vi "Periodic Tasks.vi"(8 "error in":errorcluster) -> ()   [LabVIEW 2018]
doc: "This VI runs in parallel to other robot code. It can contain as many user-defined periodic loops as you need. These can carry out PID or other sorts of timed response."
uses:
  <vilib>/Rock Robotics/Network Tables/NT Write Boolean.vi
  <vilib>/Rock Robotics/Network Tables/NT Write Number.vi
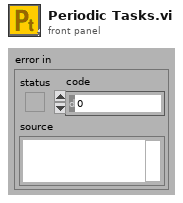
[diagram p1: front panel]
types:
  T1 = typedef "WPI_AnalogChannelDevRef.ctl" = cluster{"DevStatus":errorcluster, "Analog Channel":T2}
  T2 = typedef "FPGA_AIChannel.ctl" = enum8{"AI 0", "AI 1", "AI 2", "AI 3", "AI MXP 0", "AI MXP 1", "AI MXP 2", "AI MXP 3", "Invalid"}
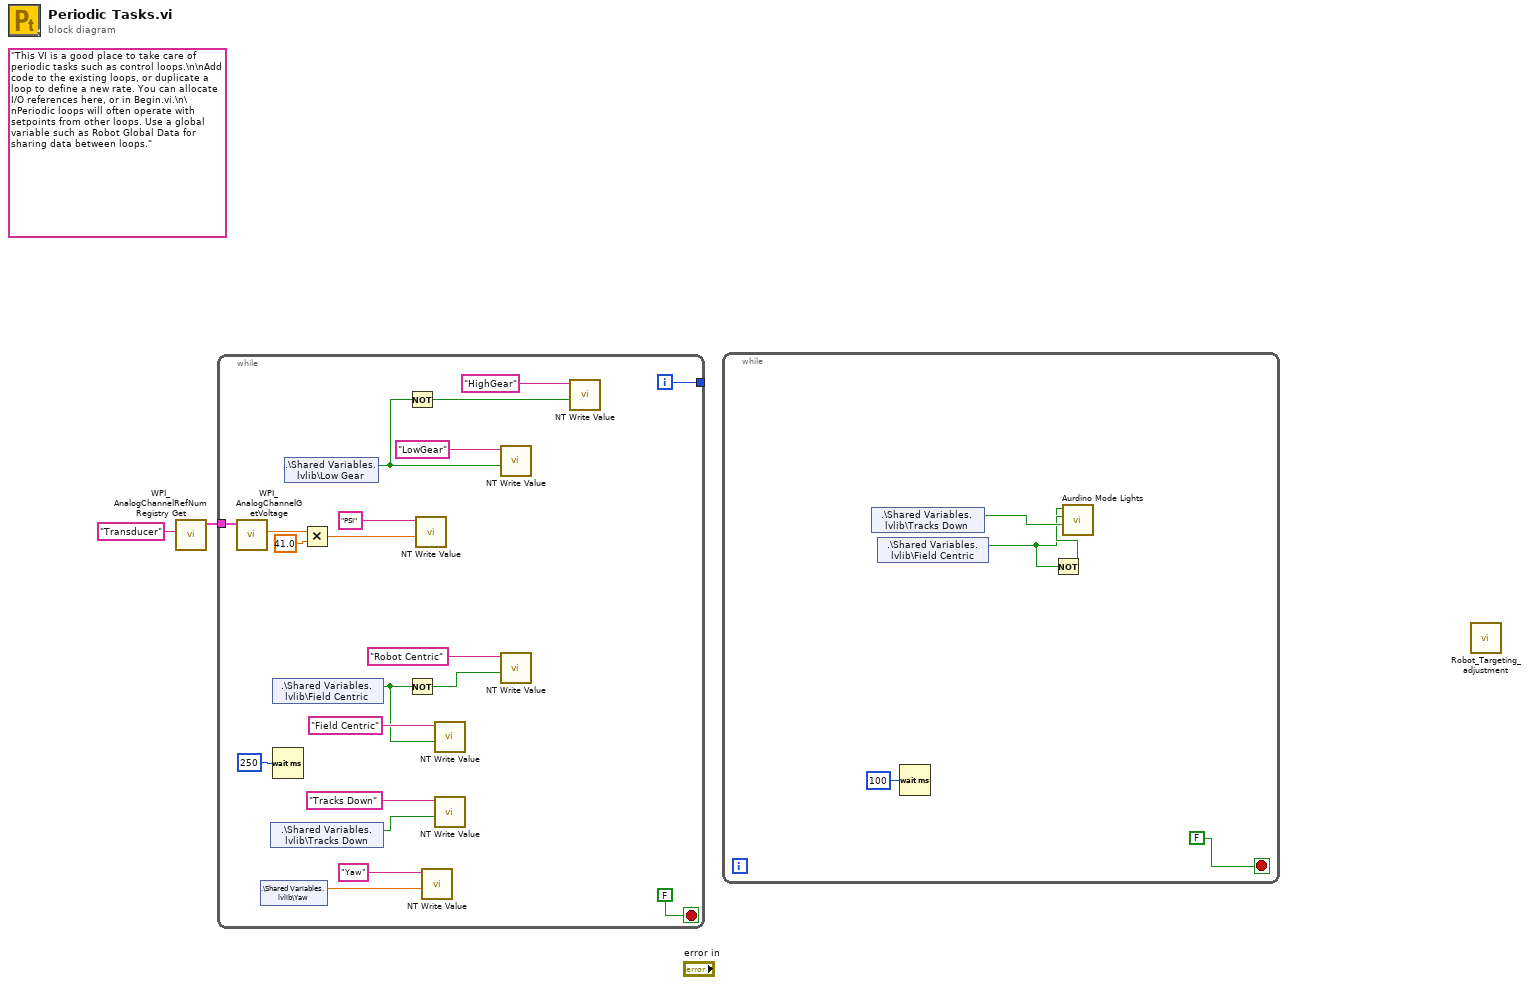
[diagram p0: block diagram]
diagram:
  (unwired) "This VI is a good place to take care of periodic tasks such as control loops.\n\nAdd code to the existing loops, or duplicate a loop to define a new rate. You can allocate I/O references here, or in Begin.vi.\n\nPeriodic loops will often operate with setpoints from other loops. Use a global variable such as Robot Global Data for sharing data between loops."
  n1 = call <vilib>:"WPI_AnalogChannelRefNum Registry Get.vi"("refnum name"="Transducer") -> ("AIDeviceRef"=w1:T1)  [unwired: 9 in, 1 out]
  n2 = while {
    tunnel: [w21] -> _
    tunnel: w1 -> [w3]
    i -> [w21]
    stop <- FALSE stop-if-true
    n3 = call <vilib>:"WPI_AnalogChannelGetVoltage.vi"("AIDeviceRef"=w3) -> ("Voltage"=w8:dbl)  [unwired: 8 in, 2 out]
    n4 = shared-variable ".\\Shared Variables.lvlib\\Yaw"() -> (w7:dbl)  [unwired: 1 in, 1 out]
    n5 = shared-variable ".\\Shared Variables.lvlib\\Tracks Down"() -> (w15:bool)  [unwired: 1 in, 1 out]
    n6 = shared-variable ".\\Shared Variables.lvlib\\Field Centric"() -> (w14:bool)  [unwired: 1 in, 1 out]
    n7 = Wait (ms)(milliseconds to wait=u32 250) -> ()  [unwired: 1 out]
    n8 = shared-variable ".\\Shared Variables.lvlib\\Low Gear"() -> (w10:bool)  [unwired: 1 in, 1 out]
    n9 = Multiply(x=w8, y=41.0) -> (x*y=w9:dbl)
    n10 = Not(x=w10) -> (.not. x?=w11:bool)
    n11 = Not(x=w14) -> (.not. x?=w16:bool)
    n12 = call-poly <vilib>:"NT Write Value.vi"("Numeric"=w9, "Name"="PSI") -> ()  [unwired: 9 in, 1 out]
    n13 = call-poly <vilib>:"NT Write Value.vi"("Numeric"=w7, "Name"="Yaw") -> ()  [unwired: 9 in, 1 out]
    n14 = call-poly <vilib>:"NT Write Value.vi"("Boolean"=w14, "Name"="Field Centric") -> ()  [unwired: 9 in, 1 out]
    n15 = call-poly <vilib>:"NT Write Value.vi"("Boolean"=w15, "Name"="Tracks Down") -> ()  [unwired: 9 in, 1 out]
    n16 = call-poly <vilib>:"NT Write Value.vi"("Boolean"=w10, "Name"="LowGear") -> ()  [unwired: 9 in, 1 out]
    n17 = call-poly <vilib>:"NT Write Value.vi"("Boolean"=w16, "Name"="Robot Centric") -> ()  [unwired: 9 in, 1 out]
    n18 = call-poly <vilib>:"NT Write Value.vi"("Boolean"=w11, "Name"="HighGear") -> ()  [unwired: 9 in, 1 out]
  }
  n19 = while {
    stop <- FALSE stop-if-true
    n20 = shared-variable ".\\Shared Variables.lvlib\\Tracks Down"() -> (w25:bool)  [unwired: 1 in, 1 out]
    n21 = shared-variable ".\\Shared Variables.lvlib\\Field Centric"() -> (w23:bool)  [unwired: 1 in, 1 out]
    n22 = Wait (ms)(milliseconds to wait=u32 100) -> ()  [unwired: 1 out]
    n23 = Not(x=w23) -> (.not. x?=w24:bool)
    n24 = call "Aurdino Mode Lights.vi"("Tracks Down"=w25, "Robot Centric"=w24, "Field Centric"=w23) -> ()  [unwired: 7 in]
  }
  n25 = call "Robot_Targeting_adjustment.vi"() -> ()  [unwired: 12 in]
